vi "Read Loads.vi"(8 "error in (no error)":errorcluster, 11 "NhRegenGridSim in":refnum<class "NhRegenGridSim.lvclass">) -> (0 "error out":errorcluster, 2 "Loads":T1[](array[typedef]), 3 "NhRegenGridSim out":refnum<class "NhRegenGridSim.lvclass">)   [LabVIEW 2014, in "AcPwrPlugins.lvlib" / "NhRegenGridSim.lvclass"]
uses:
  NhRegenGridSim.lvclass
  TypeDefs/Load.ctl
  TypeDefs/Meas.ctl
  TypeDefs/SlewRates.ctl
  TypeDefs/LoadSettings.ctl
  TypeDefs/Ranges.ctl
  NhRegenGridSim.lvclass/NhRegenGridSim.ctl
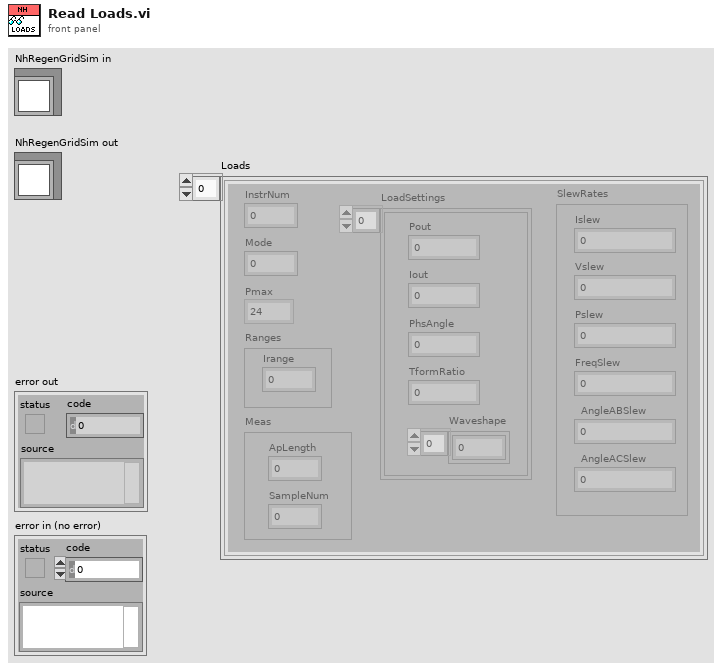
[diagram p1: front panel]
types:
  T1 = typedef "AcPwrPlugins.lvlib/NhRegenGridSim.lvclass/Load.ctl" = cluster{"Mode":u8, "InstrNum":u32, "Meas":T2, "SlewRates":T3, "LoadSettings":T4[], "Ranges":T5, "Pmax":enum16{"24 ", "48", "96"}}
  T2 = typedef "AcPwrPlugins.lvlib/NhRegenGridSim.lvclass/Meas.ctl" = cluster{"ApLength":dbl, "SampleNum":u32}
  T3 = typedef "AcPwrPlugins.lvlib/NhRegenGridSim.lvclass/SlewRates.ctl" = cluster{"Islew":dbl, "Vslew":dbl, "Pslew":dbl, "FreqSlew":dbl, "AngleABSlew":dbl, "AngleACSlew":dbl}
  T4 = typedef "AcPwrPlugins.lvlib/NhRegenGridSim.lvclass/LoadSettings.ctl" = cluster{"Pout":dbl, "Iout":dbl, "PhsAngle":dbl, "TformRatio":dbl, "Waveshape":dbl[]}
  T5 = typedef "AcPwrPlugins.lvlib/NhRegenGridSim.lvclass/Ranges.ctl" = cluster{"Irange":dbl}
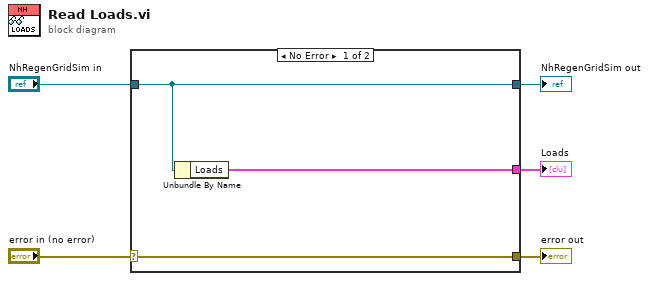
[diagram p0: block diagram]
diagram:
  n1 = case shown="No Error" "error in (no error)" {
    selector: "error in (no error)" -> [w8 w9]
    tunnel: [w8 w9] -> w4
    tunnel: [w7 w10] -> w2
    tunnel: "NhRegenGridSim in" -> [w7 w10]
    tunnel: [w6 _] -> w1
    frame No Error {
      n2 = Unbundle By Name(w7) -> ("Loads"=w6:T1[])
    }
    frame Error {
    }
  }
  "error out" <- w4
  "NhRegenGridSim out" <- w2
  "Loads" <- w1
